vi "Crypto Hash Function - LN-U8.vi"(7 "Multiplier":u8=63, 8 "error in (no error)":errorcluster, 9 "n (Hex)":string="ÿÿÿÿ", 11 "Text string":string="abcdef") -> (0 "error out":errorcluster, 2 "Hash value Hex string":string="ÿÿÿÿ", 3 "Hash Value (LI-U8)":T1=[191, 23, 168])   [LabVIEW 2013]
doc: "Generates a hash value from the input text string. Generally, for large input n values, the hash value will be have 1 less digits (base 256) than the input n value. This ensures that the hash value can properly be RSA encoded using the N value."
uses:
  User Access Type defs/Large number - U8 array.ctl
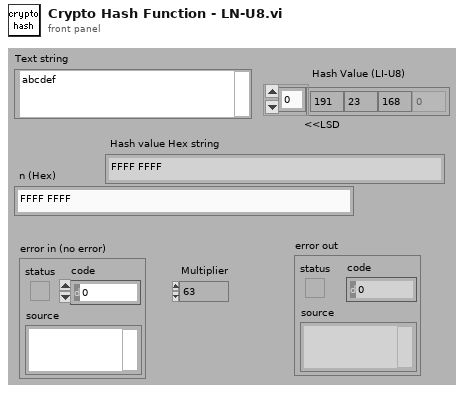
[diagram p1: front panel]
types:
  T1 = typedef "Large number - U8 array.ctl" = u8[]
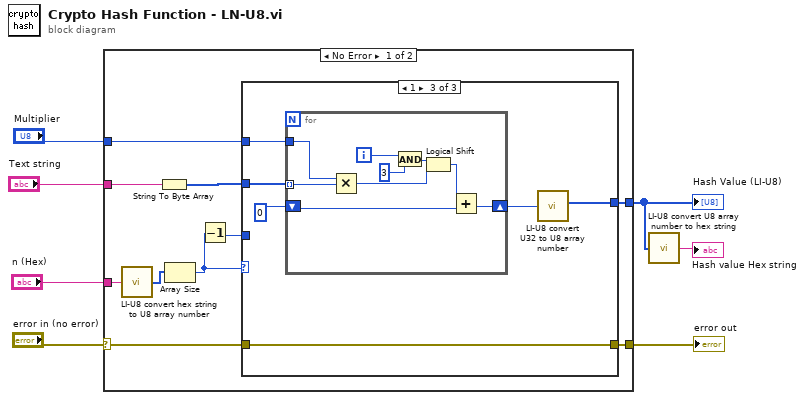
[diagram p0: block diagram]
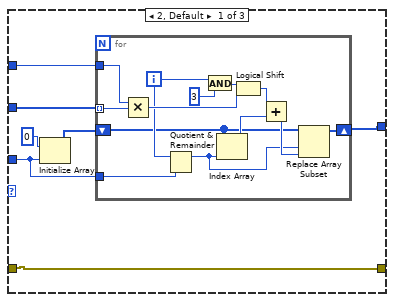
[diagram p2: hidden frame]
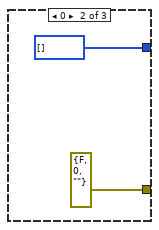
[diagram p3: hidden frame]
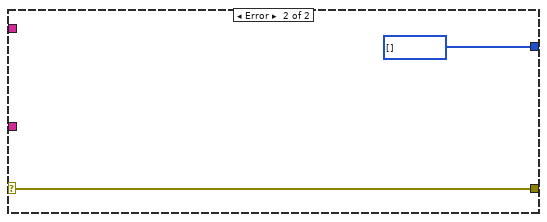
[diagram p4: hidden frame]
diagram:
  n1 = case shown="No Error" "error in (no error)" {
    selector: "error in (no error)" -> [w8 w56]
    tunnel: "Text string" -> [w17 _]
    tunnel: "n (Hex)" -> [w16 _]
    tunnel: "Multiplier" -> [w14 _]
    tunnel: [w9 w56] -> w3
    tunnel: [w13 T1 [] ("Hash Value")] -> w2
    frame No Error {
      n2 = call "LI-U8 convert hex string to U8 array number .vi"("hex string (MSD 1st)"=w16) -> ("Large number -U8"=w15:T1)  [unwired: 4 out]
      n3 = String To Byte Array(string=w17) -> (unsigned byte array=w12:u8[])
      n4 = Array Size(array=w15) -> (size(s)=w10:i32)
      n5 = Decrement(x=w10) -> (x-1=w11:i32)
      n6 = case shown="1" w10 {
        tunnel: w12 -> [w24 _ w45]
        tunnel: w11 -> [w20 _ _]
        tunnel: w14 -> [w21 _ w44]
        tunnel: [w19 u8[] [] ("Large number -U8") w41] -> w13
        tunnel: w8 -> [w18 _ w40]
        tunnel: [w18 errorcluster {"status"=FALSE, "code"=0, "source"=""} ("error IO") w40] -> w9
        frame 2, Default {
          n7 = Initialize Array(u8 0 ("element"), w20) -> (w22:u8[])
          n8 = for {
            tunnel: w24 -> [w33] mode=indexing
            shift-right: [w25] -> w19
            shift-left: w22 -> [w27]
            tunnel: w21 -> [w32]
            tunnel: w20 -> [w30]
            i -> [w31]
            n9 = Multiply(x=w32, y=w33) -> (x*y=w35:u8)
            n10 = Quotient & Remainder(x=w31, y=w30) -> (x-y*floor(x/y)=w26:i32)  [unwired: 1 out]
            n11 = And(x=w31, y=3) -> (x .and. y?=w36:i32)
            n12 = Index Array(array=w27, index=w26) -> (element=w29:u8)
            n13 = Logical Shift(y=w36, x=w35) -> (x << y=w34:u8)
            n14 = Add(x=w34, y=w29) -> (x+y=w28:u8)
            n15 = Replace Array Subset(array=w27, new element=w28, index=w26) -> (w25:u8[])
          }
        }
        frame 0 {
        }
        frame 1 {
          n16 = for {
            tunnel: w45 -> [w49] mode=indexing
            shift-right: [w46] -> w42
            shift-left: u32 0 ("element") -> [w47]
            tunnel: w44 -> [w48]
            i -> [w54]
            n17 = Multiply(x=w48, y=w49) -> (x*y=w51:u8)
            n18 = And(x=w54, y=3) -> (x .and. y?=w52:i32)
            n19 = Logical Shift(y=w52, x=w51) -> (x << y=w50:u8)
            n20 = Add(x=w50, y=w47) -> (x+y=w46:u32)
          }
          n21 = call "LI-U8 convert U32 to U8 array number.vi"("U32"=w42) -> ("Large number -U8"=w41:T1)  [unwired: 4 out]
        }
      }
    }
    frame Error {
    }
  }
  "Hash Value (LI-U8)" <- w2
  "error out" <- w3
  n22 = call "LI-U8 convert U8 array number to hex string.vi"("Large number -U8"=w2) -> ("hex string (MSD 1st)"=→"Hash value Hex string":string)  [unwired: 4 out]
